vi "Copilot States.vi"(9 "Drive Metrics in":T2) -> (1 "Drive Metrics out":T2)   [LabVIEW 2015]
uses:
  Drive Metrics.ctl
  Drive States.ctl
  Copilot States.ctl
  <vilib>/Rock Robotics/WPI/CAN/TalonSRX/WPI_CANTalonSRX_APIControlMode.ctl
  Support/Global Objects.vi
panel:
  out "Waveforms":T1(graph)
  in  "Flywheel Power":dbl
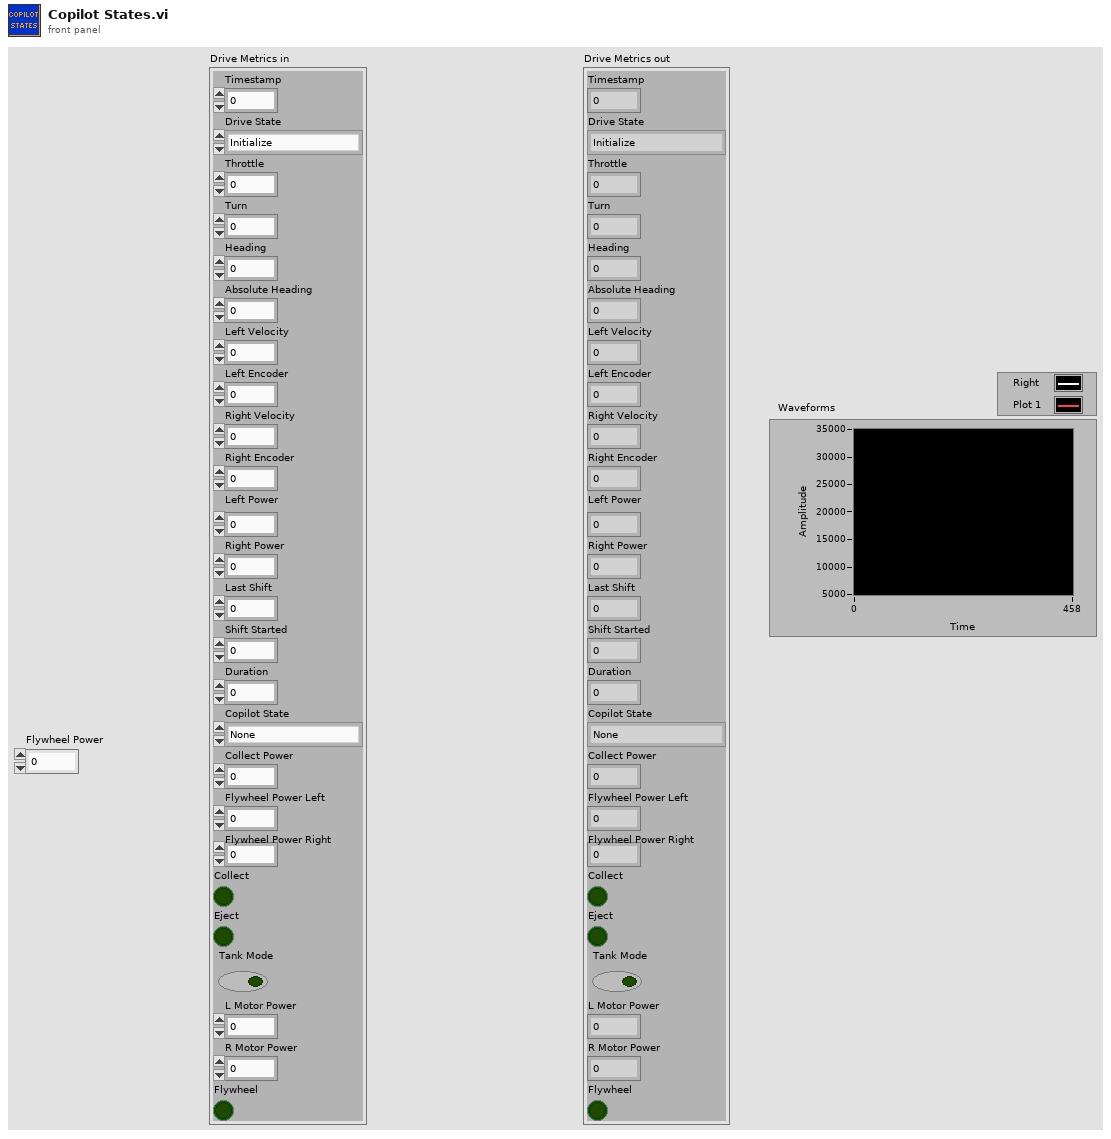
[diagram p1: front panel]
types:
  T1 = cluster{"Sensor Velocity":dbl, "Sensor Velocity":dbl}
  T2 = typedef "Drive Metrics.ctl" = cluster{"Timestamp":u32, "Drive State":T3, "Throttle":dbl, "Turn":dbl, "Heading":dbl, "Absolute Heading":dbl, "Left Velocity":dbl, "Left Encoder":dbl, "Right Velocity":dbl, "Right Encoder":dbl, "Left Power":dbl, "Right Power":dbl, "Last Shift":u32, "Shift Started":u32, "Duration":i64, "Copilot State":T4, "Collect Power":dbl, "Flywheel Power Left":dbl, "Flywheel Power Right":dbl, "Collect":bool, "Eject":bool, "Tank Mode":bool, "L Motor Power":dbl, "R Motor Power":dbl, "Flywheel":bool}
  T3 = typedef "Drive States.ctl" = enum16{"Initialize", "Low Gear", "Up Shift Begin", "Up Shifting", "Up Shift Delay", "High Gear", "Down Shift Begin", "Down Shifting", "Down Shift Delay"}
  T4 = typedef "Copilot States.ctl" = enum16{"None", "Lift collector", "Boulder to shooter", "Lifting collector", "Lifted Collector", "Collected", "Collecting", "Ejecting", "Dropping arm", "Boulder ready", "Shooter to angle", "Flywheel spin up", "Drop arm", "Flywheel ready"}
  T5 = typedef "WPI_CANTalonSRX_APIControlMode.ctl" = enum8{"Percent VBus", "Speed", "Position", "Slave", "Unchanged / Invalid", "Voltage Compensation", "Current", "Motion Profile"}
  T6 = typedef "Motor Typedef.ctl" = cluster{"Motor1":T7, "Last Motor Power":dbl}
  T7 = typedef "WPI_MotorControlDeviceRef.ctl" = cluster{"DeviceStatus":errorcluster, "Type":T8, "PWM":cluster{"PWM Channel":T9, "DeadBand":T10}, "CAN":cluster{"Device Number":u8, "Control Mode":T11, "Semaphore":T12, "Max Vout":dbl, "TalonSRX Control Mode":T5}, "Invert":bool}
  T8 = typedef "WPI_MotorControlType.ctl" = enum16{"PWM", "CAN", "CANTalonSRX"}
  T9 = typedef "FPGA_DIOPWMChannel.ctl" = enum8{"PWM 0", "PWM 1", "PWM 2", "PWM 3", "PWM 4", "PWM 5", "PWM 6", "PWM 7", "PWM 8", "PWM 9", "PWM MXP 0", "PWM MXP 1", "PWM MXP 2", "PWM MXP 3", "PWM MXP 4", "PWM MXP 5", "PWM MXP 6", "PWM MXP 7", "PWM MXP 8", "PWM MXP 9", "Invalid"}
  T10 = typedef "WPI_PWMDeadband.ctl" = cluster{"Name":string, "maxPositivePwm":i32, "minPositivePwm":i32, "centerPwm":i32, "maxNegativePwm":i32, "minNegativePwm":i32, "angularRange":u16}
  T11 = typedef "WPI_CANJaguar_ControlMode.ctl" = enum8{"Percent VBus", "Current", "Speed", "Position", "Voltage"}
  T12 = typedef "Semaphore RefNum" = refnum<k1>
  T13 = typedef "Configuration.ctl" = cluster{"Throttle Dead Zone":dbl, "Throttle Ramp Rate":dbl, "Turn Dead Zone":dbl, "Auton":cluster{"Motion Plan P":dbl, "Motion Plan I":dbl, "Motion Plan D":dbl}, "Auto Upshift Enabled":bool, "Upshift Min Throttle":dbl, "Upshift Min Velocity":dbl, "Min time before upshift":dbl, "Shift Throttle Detent":u32, "Min time before downshift":dbl, "Turn PID":cluster{"Motion Plan P":dbl, "Motion Plan I":dbl, "Motion Plan D":dbl}, "Auto Coast Downshift":bool, "Downshift Coast Max Vel":dbl, "Downshift Coast Throttle Epsilon":dbl, "Left Motor Calibration":dbl, "Right Motor Calibration":dbl, "Tank Mode":bool, "Shooter PID":cluster{"Shooter  P":dbl, "Shooter  I":dbl, "Shooter  D":dbl}}
  T14 = typedef "WPI_CANTalonSRX_GlobalStatus.ctl" = cluster{"Applied Throttle":dbl, "Module Enabled":bool, "CAN Error":errorcluster, "Closed Loop Error":dbl, "Forward Limit Switch Closed":bool, "Reverse Limit Switch Closed":bool, "Sensor Position":dbl, "Sensor Velocity":dbl, "Current":dbl, "Sticky Fault - Over Temp":bool, "Sticky Fault - Under Voltage":bool, "Sticky Fault - Forward Limit":bool, "Sticky Fault - Reverse Limit":bool, "Sticky Fault - Forward Soft Limit":bool, "Sticky Fault - Reverse Soft Limit":bool, "Brake is Enabled":bool, "Encoder Position":dbl, "Encoder Velocity":dbl, "Encoder Index Count":dbl, "Encoder A Pin State":bool, "Encoder B Pin State":bool, "Encoder Index Pin State":bool, "Analog In":dbl, "Analog In Velocity":dbl, "Temperature (C)":dbl, "Battery Voltage":dbl, "Control 5 Is Supported":bool, "Current Profile Slot Select":dbl, "Pos Div 8":bool, "Vel Div 4":bool, "Pulse Width Position":i32, "Pulse Width Velocity":i32, "Pulse Width Rise To Rise (us)":i32, "Pulse Width Rise To Fall (us)":i32, "Mot Prof Active Is Under Run":bool, "Mot Prof Active Has Under Run":bool, "Mot Prof Active Is Last":bool, "Mot Prof Active Velocity Only":bool, "Mot Prof Active Is Valid":bool, "Mot Prof Buffer Is Full":bool, "Mot Prof Active Profile Slot Select":i32, "Mot Prof NextID":i32, "Mot Prof Count":i32, "Mot Prof Active Velocity":dbl, "Mot Prof Active Position":dbl, "Mot Prof Output Enable":i32}
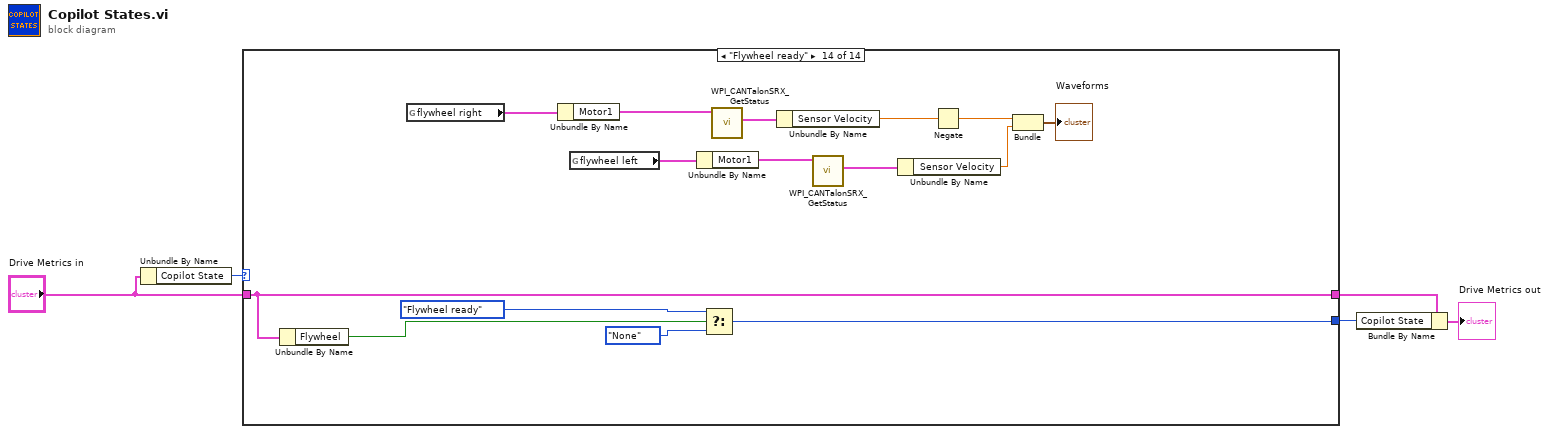
[diagram p0: block diagram]
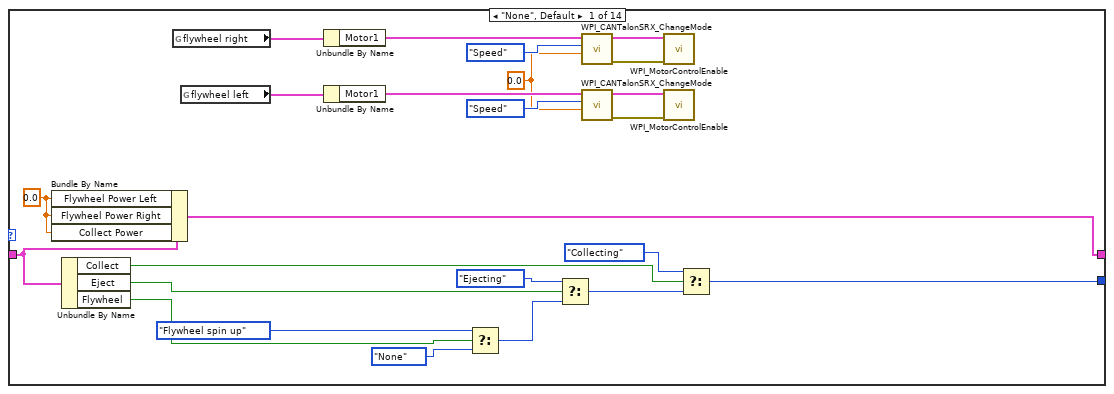
[diagram p2: hidden frame]
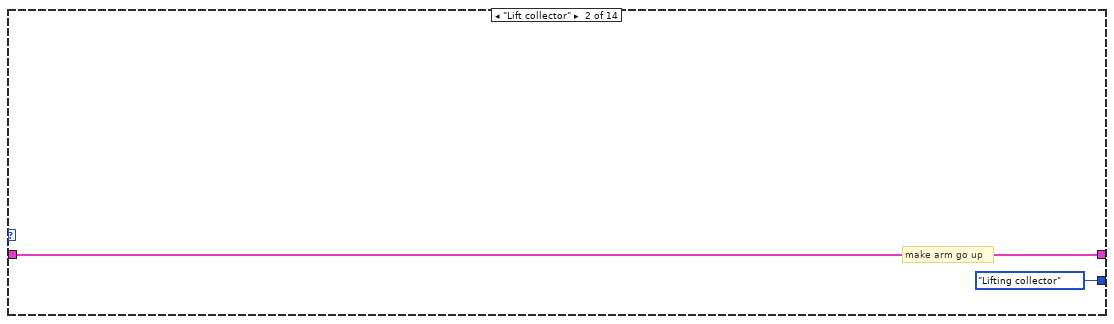
[diagram p3: hidden frame]
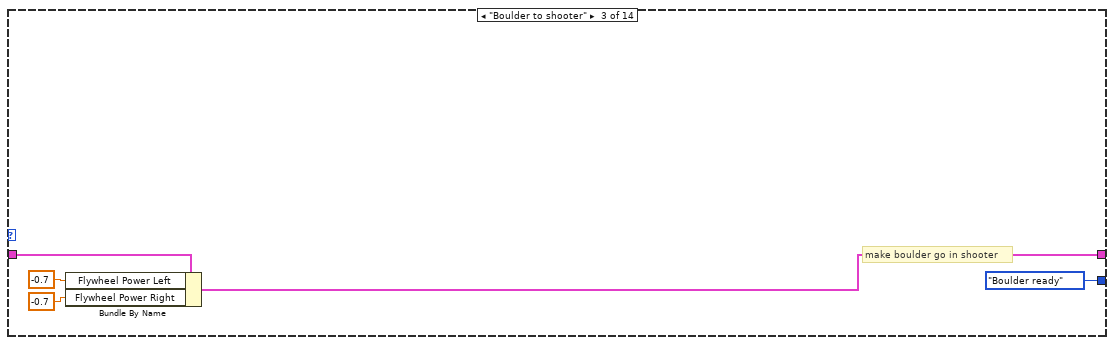
[diagram p4: hidden frame]
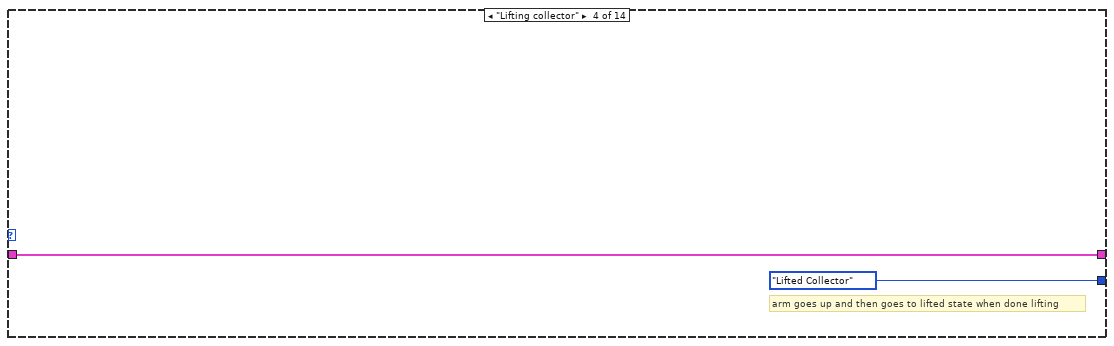
[diagram p5: hidden frame]
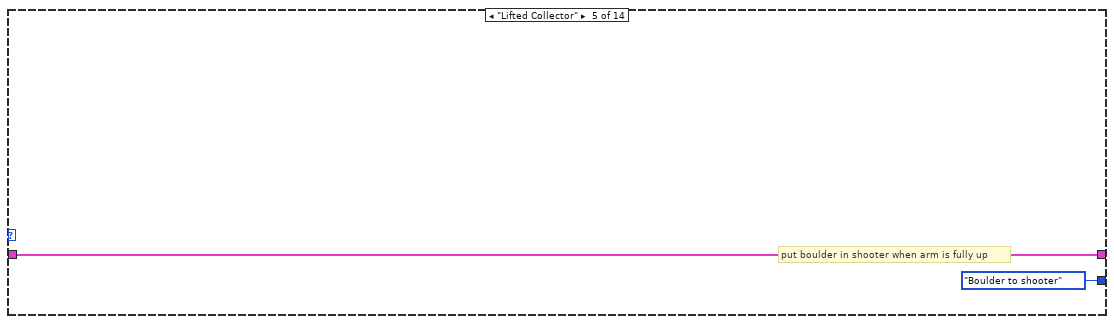
[diagram p6: hidden frame]
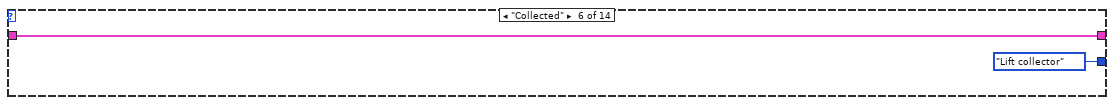
[diagram p7: hidden frame]
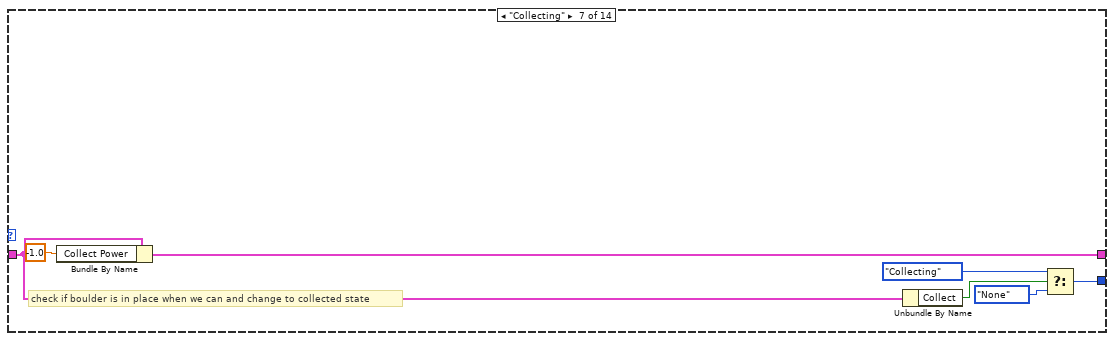
[diagram p8: hidden frame]
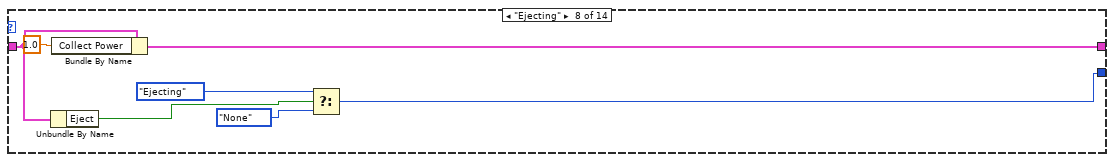
[diagram p9: hidden frame]
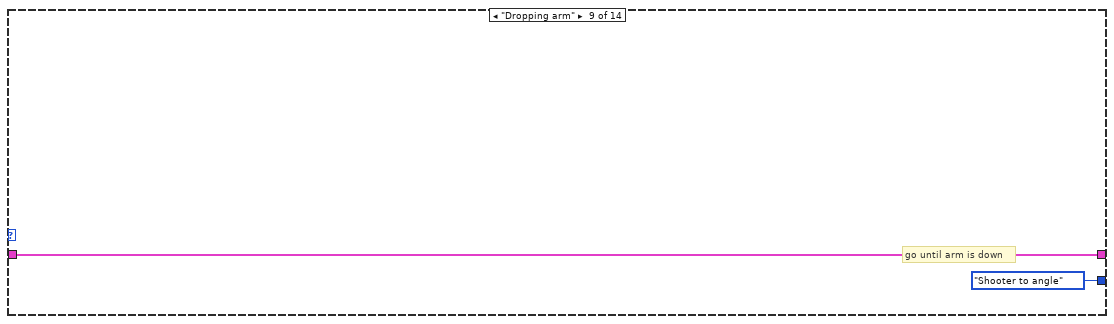
[diagram p10: hidden frame]
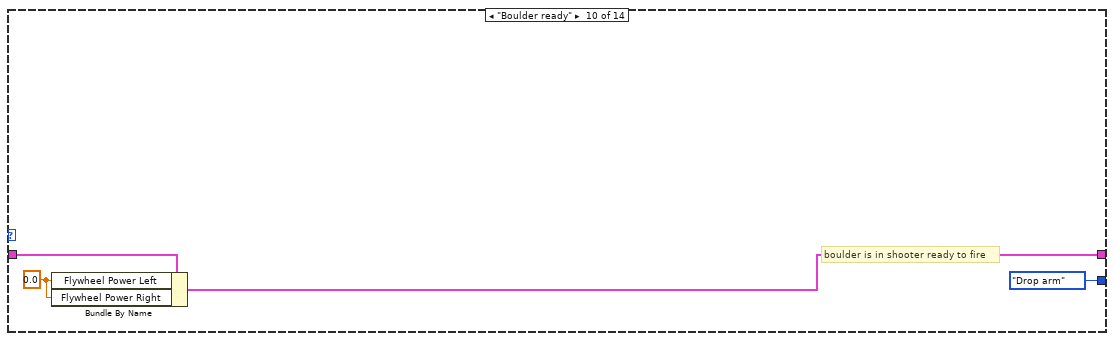
[diagram p11: hidden frame]
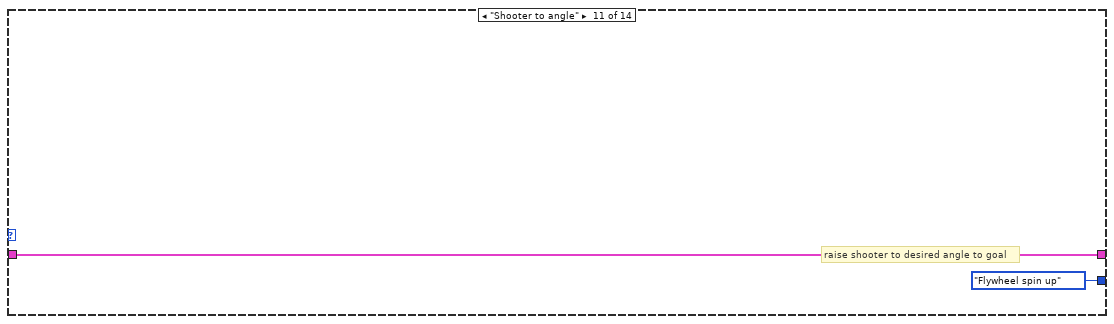
[diagram p12: hidden frame]
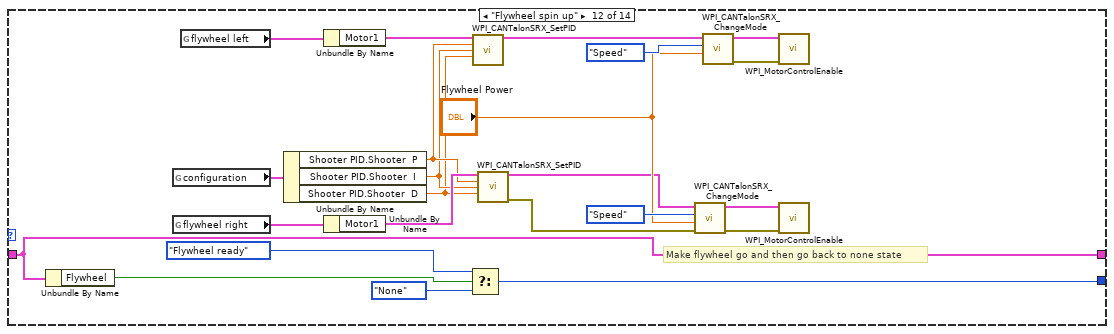
[diagram p13: hidden frame]
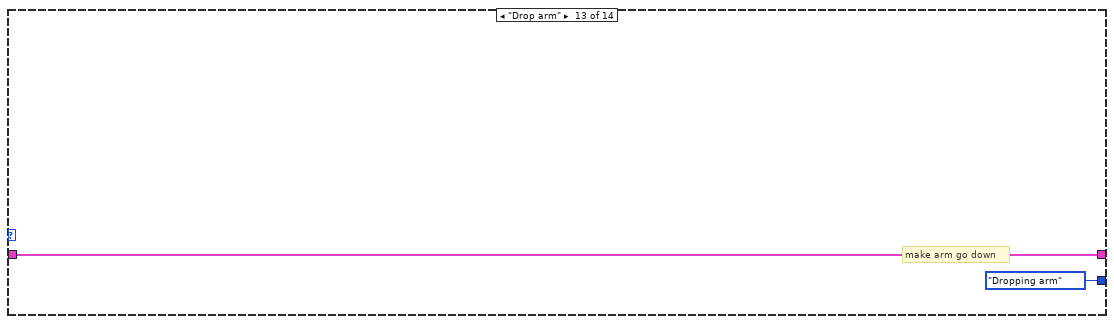
[diagram p14: hidden frame]
diagram:
  n1 = Unbundle By Name("Drive Metrics in") -> ("Copilot State"=w4:T4)
  n2 = case shown="\"Flywheel ready\"" w4 {
    tunnel: "Drive Metrics in" -> [w23 w31 w34 w38 w40 w42 w47 w51 w58 w62 w64 w84 w89 w101]
    tunnel: [w22 w31 w35 w38 w40 w42 w48 w55 w58 w60 w64 w84 w89 w101] -> w3
    tunnel: [w27 Copilot_States."Lifting collector" ("Copilot State") Copilot_States."Boulder ready" ("Copilot State") Copilot_States."Lifted Collector" ("Copilot State") Copilot_States."Boulder to shooter" ("Copilot State") Copilot_States."Lift collector" ("Copilot State") w44 w50 Copilot_States."Shooter to angle" ("Copilot State") Copilot_States."Drop arm" ("Copilot State") Copilot_States."Flywheel spin up" ("Copilot State") w85 Copilot_States."Dropping arm" ("f") w100] -> w1
    frame "None", Default {
      w7 = 0.0 ("Flywheel Power 2")
      w21 = 0.0 ("Collect Power")
      n3 = Bundle By Name(cluster=w23, "Flywheel Power Left"=w21, "Flywheel Power Right"=w21, "Collect Power"=w21) -> (w22:T2)
      n4 = Unbundle By Name(w23) -> ("Collect"=w29:bool, "Eject"=w24:bool, "Flywheel"=w20:bool)
      n5 = global read "Global Objects.vi" "flywheel right"() -> (w12:T6)
      n6 = global read "Global Objects.vi" "flywheel left"() -> (w17:T6)
      n7 = Unbundle By Name(w12) -> ("Motor1"=w11:T7)
      n8 = Unbundle By Name(w17) -> ("Motor1"=w16:T7)
      n9 = Select(t=Copilot_States."Flywheel spin up" ("Copilot State"), s=w20, f=Copilot_States."None") -> (s? t:f=w18:T4)
      n10 = Select(t=Copilot_States."Ejecting" ("Copilot State"), s=w24, f=w18) -> (s? t:f=w25:T4)
      n11 = call <vilib>:"WPI_CANTalonSRX_ChangeMode.vi"("Output"=w7, "Control Mode"=WPI_CANTalonSRX_APIControlMode."Speed", "CAN Talon SRX Ref"=w11) -> ("error out"=w9:errorcluster, "CAN Talon SRX Ref"=w10:T7)  [unwired: 7 in]
      n12 = call <vilib>:"WPI_CANTalonSRX_ChangeMode.vi"("Output"=w7, "Control Mode"=WPI_CANTalonSRX_APIControlMode."Speed", "CAN Talon SRX Ref"=w16) -> ("error out"=w14:errorcluster, "CAN Talon SRX Ref"=w15:T7)  [unwired: 7 in]
      n13 = call <vilib>:"WPI_MotorControlEnable.vi"("error in (no error)"=w9, "CAN MotorDevRef"=w10) -> ()  [unwired: 8 in, 2 out]
      n14 = call <vilib>:"WPI_MotorControlEnable.vi"("error in (no error)"=w14, "CAN MotorDevRef"=w15) -> ()  [unwired: 8 in, 2 out]
      n15 = Select(t=Copilot_States."Collecting" ("Copilot State"), s=w29, f=w25) -> (s? t:f=w27:T4)
    }
    frame "Lift collector" {
      # "make arm go up"
    }
    frame "Boulder to shooter" {
      # "make boulder go in shooter"
      n16 = Bundle By Name(cluster=w34, "Flywheel Power Left"=-0.7 ("Throttle"), "Flywheel Power Right"=-0.7 ("Throttle")) -> (w35:T2)
    }
    frame "Lifting collector" {
      # "arm goes up and then goes to lifted state when done lifting"
    }
    frame "Lifted Collector" {
      # "put boulder in shooter when arm is fully up"
    }
    frame "Collected" {
    }
    frame "Collecting" {
      # "check if boulder is in place when we can and change to collected state"
      n17 = Bundle By Name(cluster=w47, "Collect Power"=-1.0) -> (w48:T2)
      n18 = Unbundle By Name(w47) -> ("Collect"=w46:bool)
      n19 = Select(t=Copilot_States."Collecting" ("Copilot State"), s=w46, f=Copilot_States."None" ("Copilot State")) -> (s? t:f=w44:T4)
    }
    frame "Ejecting" {
      n20 = Unbundle By Name(w51) -> ("Eject"=w52:bool)
      n21 = Bundle By Name(cluster=w51, "Collect Power"=1.0) -> (w55:T2)
      n22 = Select(t=Copilot_States."Ejecting" ("Copilot State"), s=w52, f=Copilot_States."None" ("Copilot State")) -> (s? t:f=w50:T4)
    }
    frame "Dropping arm" {
      # "go until arm is down"
    }
    frame "Boulder ready" {
      w61 = 0.0 ("Flywheel Power Left")
      # "boulder is in shooter ready to fire"
      n23 = Bundle By Name(cluster=w62, "Flywheel Power Left"=w61, "Flywheel Power Right"=w61) -> (w60:T2)
    }
    frame "Shooter to angle" {
      # "raise shooter to desired angle to goal"
    }
    frame "Flywheel spin up" {
      # "Make flywheel go and then go back to none state"
      n24 = Unbundle By Name(w84) -> ("Flywheel"=w86:bool)
      n25 = global read "Global Objects.vi" "configuration"() -> (w65:T13)
      n26 = global read "Global Objects.vi" "flywheel right"() -> (w79:T6)
      n27 = global read "Global Objects.vi" "flywheel left"() -> (w83:T6)
      n28 = Unbundle By Name(w65) -> ("Shooter PID.Shooter  P"=w68:dbl, "Shooter PID.Shooter  I"=w67:dbl, "Shooter PID.Shooter  D"=w66:dbl)
      n29 = Unbundle By Name(w83) -> ("Motor1"=w70:T7)
      n30 = Unbundle By Name(w79) -> ("Motor1"=w73:T7)
      n31 = Select(t=Copilot_States."Flywheel ready" ("f"), s=w86, f=Copilot_States."None") -> (s? t:f=w85:T4)
      n32 = call <vilib>:"WPI_CANTalonSRX_SetPID.vi"("CAN Talon SRX Ref"=w70, "P"=w68, "I"=w67, "D"=w66) -> ("CAN Talon SRX Ref"=w69:T7)  [unwired: 10 in, 1 out]
      n33 = call <vilib>:"WPI_CANTalonSRX_SetPID.vi"("CAN Talon SRX Ref"=w73, "P"=w68, "I"=w67, "D"=w66) -> ("CAN Talon SRX Ref"=w72:T7, "error out"=w71:errorcluster)  [unwired: 10 in]
      n34 = call <vilib>:"WPI_CANTalonSRX_ChangeMode.vi"("error in (no error)"=w71, "Output"="Flywheel Power", "Control Mode"=WPI_CANTalonSRX_APIControlMode."Speed", "CAN Talon SRX Ref"=w72) -> ("error out"=w77:errorcluster, "CAN Talon SRX Ref"=w78:T7)  [unwired: 6 in]
      n35 = call <vilib>:"WPI_CANTalonSRX_ChangeMode.vi"("Output"="Flywheel Power", "Control Mode"=WPI_CANTalonSRX_APIControlMode."Speed", "CAN Talon SRX Ref"=w69) -> ("error out"=w81:errorcluster, "CAN Talon SRX Ref"=w82:T7)  [unwired: 7 in]
      n36 = call <vilib>:"WPI_MotorControlEnable.vi"("error in (no error)"=w81, "CAN MotorDevRef"=w82) -> ()  [unwired: 8 in, 2 out]
      n37 = call <vilib>:"WPI_MotorControlEnable.vi"("error in (no error)"=w77, "CAN MotorDevRef"=w78) -> ()  [unwired: 8 in, 2 out]
    }
    frame "Drop arm" {
      # "make arm go down"
    }
    frame "Flywheel ready" {
      n38 = Unbundle By Name(w101) -> ("Flywheel"=w102:bool)
      n39 = global read "Global Objects.vi" "flywheel right"() -> (w99:T6)
      n40 = Unbundle By Name(w99) -> ("Motor1"=w98:T7)
      n41 = global read "Global Objects.vi" "flywheel left"() -> (w96:T6)
      n42 = Unbundle By Name(w96) -> ("Motor1"=w95:T7)
      n43 = Select(t=Copilot_States."Flywheel ready" ("f"), s=w102, f=Copilot_States."None") -> (s? t:f=w100:T4)
      n44 = call <vilib>:"WPI_CANTalonSRX_GetStatus.vi"("CAN Talon SRX Ref"=w98) -> ("Talon SRX Status"=w97:T14)  [unwired: 8 in, 2 out]
      n45 = Unbundle By Name(w97) -> ("Sensor Velocity"=w91:dbl)
      n46 = call <vilib>:"WPI_CANTalonSRX_GetStatus.vi"("CAN Talon SRX Ref"=w95) -> ("Talon SRX Status"=w94:T14)  [unwired: 8 in, 2 out]
      n47 = Unbundle By Name(w94) -> ("Sensor Velocity"=w93:dbl)
      n48 = Negate(x=w91) -> (-x=w90:dbl)
      n49 = Bundle(w90, "Sensor Velocity"=w93) -> (→"Waveforms":cluster{dbl, "Sensor Velocity":dbl})  [unwired: 1 in]
    }
  }
  n50 = Bundle By Name(cluster=w3, "Copilot State"=w1) -> (→"Drive Metrics out":T2)
